vi "Read Image path.vi"(8 "error in (no error)":errorcluster, 11 "MessageBox.lvclass in":refnum<class "MessageBox.lvclass">) -> (0 "error out":errorcluster, 2 "Image path":path, 3 "MessageBox.lvclass out":refnum<class "MessageBox.lvclass">)   [LabVIEW 2012, in "MessageBox.lvlib" / "MessageBox.lvclass"]
uses:
  MessageBox.lvclass
  MessageBox.lvclass/MessageBox.ctl
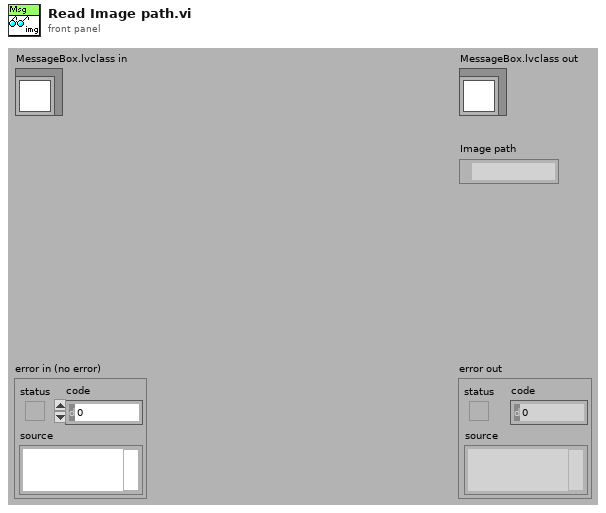
[diagram p1: front panel]
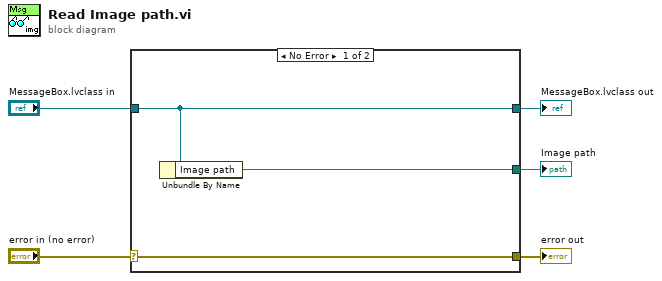
[diagram p0: block diagram]
diagram:
  n1 = case shown="No Error" "error in (no error)" {
    selector: "error in (no error)" -> [w8 w9]
    tunnel: [w8 w9] -> w4
    tunnel: [w7 w10] -> w2
    tunnel: "MessageBox.lvclass in" -> [w7 w10]
    tunnel: [w6 _] -> w1
    frame No Error {
      n2 = Unbundle By Name(w7) -> ("Image path"=w6:path)
    }
    frame Error {
    }
  }
  "error out" <- w4
  "MessageBox.lvclass out" <- w2
  "Image path" <- w1
